vi "Count Adjust.vi"(9 "Button Cluster":T1, 10 "Axes":dbl[](array[numeric])) -> ()   [LabVIEW 2014]
uses:
  Real-Life Controls/Button Cluster.ctl
  Common Code/Change Detect Boolean.vi
  Robot Global Data.vi
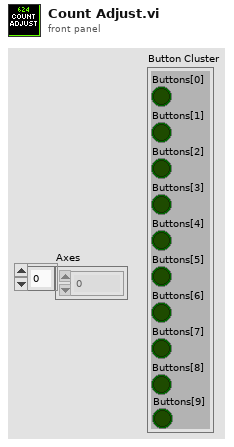
[diagram p1: front panel]
types:
  T1 = typedef "Button Cluster.ctl" = cluster{"Buttons[0]":bool, "Buttons[1]":bool, "Buttons[2]":bool, "Buttons[3]":bool, "Buttons[4]":bool, "Buttons[5]":bool, "Buttons[6]":bool, "Buttons[7]":bool, "Buttons[8]":bool, "Buttons[9]":bool}
  T2 = enum16{"0", "1", "2", "3", "4", "5", "6", "7", "8", "9", "A", "B", "C", "D", "E", "F", "G", "H", "I", "J", "K", "L", "M", "N", "O", "P", "Q", "R", "S", "T", "U", "V", "W", "X", "Y", "Z", "F1", "F2", "F3", "F4", "F5", "F6", "F7", "F8", "F9", "F10", "F11", "F12", "F13", "F14", "F15", "ADD", "BACK", "BACKSLASH", "CAPITAL", "COMMA", "DECIMAL", "DELETE", "DIVIDE", "DOWN", "END", "EQUALS", "ESCAPE", "GRAVE (`)", "HOME", "INSERT", "LBRACKET", "LCONTROL", "LEFT", "L ALT", "LSHIFT", "LWIN", "MINUS", "MULTIPLY", "NEXT", "NUMLOCK", "NUMPAD_0", "NUMPAD_1", "NUMPAD_2", "NUMPAD_3", "NUMPAD_4", "NUMPAD_5", "NUMPAD_6", "NUMPAD_7", "NUMPAD_8", "NUMPAD_9", "PAUSE", "PERIOD", "PRIOR (PG UP)", "RBRACKET", "RCONTROL", "RETURN", "RIGHT", "R ALT", "RSHIFT", "RWIN", "SCROLL", "SEMICOLON", "SLASH", "SPACE", "SUBTRACT", "TAB", "UP", "ENTER (num pad)", "' (quote)"}
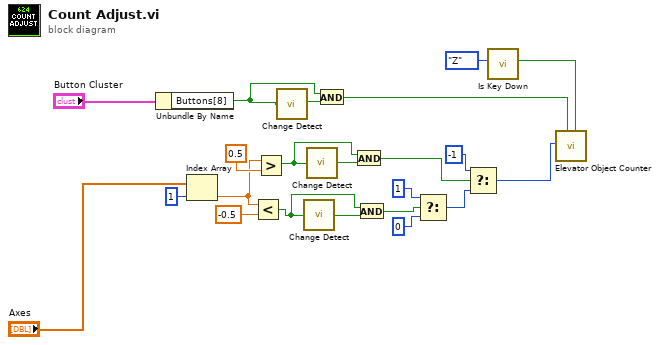
[diagram p0: block diagram]
diagram:
  n1 = Unbundle By Name("Button Cluster") -> ("Buttons[8]"=w3:bool)
  n2 = Index Array(array="Axes", index=1) -> (element=w6:dbl)
  n3 = Less?(x=w6, y=-0.5) -> (x < y?=w11:bool)
  n4 = Greater?(x=w6, y=0.5 ("x")) -> (0:w9:bool)
  n5 = call-poly "Change Detect.vi"("In"=w3) -> ("Changed?"=w18:bool)
  n6 = call-poly "Change Detect.vi"("In"=w11) -> ("Changed?"=w10:bool)
  n7 = call-poly "Change Detect.vi"("In"=w9) -> ("Changed?"=w8:bool)
  n8 = And(x=w3, y=w18) -> (x .and. y?=w19:bool)
  n9 = And(x=w9, y=w8) -> (x .and. y?=w16:bool)
  n10 = And(x=w11, y=w10) -> (x .and. y?=w12:bool)
  n11 = Select(t=1, s=w12, f=0) -> (s? t:f=w15:i32)
  n12 = Select(t=-1, s=w16, f=w15) -> (s? t:f=w20:i32)
  n13 = call "Is Key Down.vi"("Key"=T2."Z") -> ("Key Down?"=w2:bool)  [unwired: 10 in]
  n14 = call "Elevator Object Counter.vi"("Clear Stack?"=w2, "Toggle Trashcan?"=w19, "Tote Delta"=w20) -> ()  [unwired: 7 in, 2 out]
